vi "GettingStarted.vi"() -> ()   [LabVIEW 2014, in "Sixpack - Driver.lvlib"]
uses:
  Sixpack - Driver.lvlib
  Activity.ctl
  MotorParameter_P5.ctl
  MotorParameter_P6.ctl
  Current.ctl
panel:
  out "polling chart":u32(graph)
  out "error chart":i8(graph)
  in  "UnitAddress":u16=1
  out "error out":errorcluster
  out "StopFlag":bool
  out "CurrentActivity":T1
  out "CurrentPosition":i32 caption="Steps"
  out "Polling Time":u32 caption="msec"
  in  "Stop":bool
  in  "Tab Control":T2(tab)=enum."Interface"
  in  "Stop Motors":bool
  in  "Motors":T3
  in  "SetActualPos":bool
  in  "ActualPosition":u8 caption="Steps"
  in  "TargetPosition":i32 caption="Steps"
  in  "Ramp":bool
  out "TtlIo1":u8
  out "RefInput":bool
  out "AnalogInput":dbl(graph)
  out "AllInputs":T4
  in  "AcceleratingCurrent(100%)":T5
  in  "RunningCurrent(75%)":T5=enum."75%"
  in  "StandingCurrent(50%)":T5=enum."50%"
  in  "PowerDownCurrent(0%)":T5=enum."0%"
  in  "MotNr (0+1)":enum8{"0+1", "2+3", "4+5"}(ring)
  in  "Imax (0-800mA)":dbl=400.0
  in  "PowerDownDelay(500)":u16=500
  in  "SetCurrent":bool
  out "FMin":dbl
  out "FStart":dbl
  out "Fmax":dbl
  in  "VMax(511)":u16=511
  in  "AMax(128)":u16=128
  in  "Div(2)":u8=2
  in  "VMin(4)":u16=4
  in  "VStart(5)":u16=5
  in  "ClockDivider (5)":u8=5
  in  "SetVelocity":bool
  in  "PosLimit(6400)":u32=6400
  in  "SetMotorParameter":bool
  in  "P6 Bits":T6={"MT_OPTIMIZEWAY"=FALSE, "MT_FASTREF"=TRUE, "MT_MECHREF"=FALSE, "MT_DELAYTESTNULL"=TRUE, "MT_STOPSOFT"=FALSE, "MT_STOPNOREF"=FALSE, "MT_NULLPOSITIVE"=FALSE, "MUT_STOPFULSTEPS"=FALSE}
  in  "P5 Bits":T7={"MT_PI"=FALSE, "MT_ROTARY"=FALSE, "MT_AUTONULLCMD"=FALSE, "MT_TESTNULL"=FALSE, "MT_NULLLEFT"=FALSE, "MT_NULLCENTRE"=TRUE, "MT_STOPNULL"=FALSE, "MT_FILTERSWITCH"=TRUE}
  in  "SetLimits":bool
  in  "MaxRight(1023)":u16=1023
  in  "MinLeft(0)":u16
  in  "StartRefSearch":bool
  in  "Set ReferenceSwitchConfig":bool
  in  "Margin(0)":u16
  in  "TestNullRange(240)":u16
  in  "NullOffset(0)":i32
  out "FRefMax":dbl
  in  "DebouncingTime (22ms)":u8 format="%x"
  in  "VRefMax(100)":u16=100
  in  "Set RefSearchParameters":bool
  in  "Reset":bool
  out "SerialNumber":u16
  out "Temperature":i16 caption="Celsius"
  out "ResetFlag":bool
  out "FirmwareRevision":u8
  in  "OpenPort":bool
  out "Handle":i32=-1
  in  "BaudRate (19200)":enum32{"9600", "19200", "38400", "57600"}(ring)=enum."57600"
  in  "COM Port (COM1)":T8(ring)=enum."COM2"
  in  "MotNr":u8=1
  in  "PdcInt":i32=100 caption="msec"
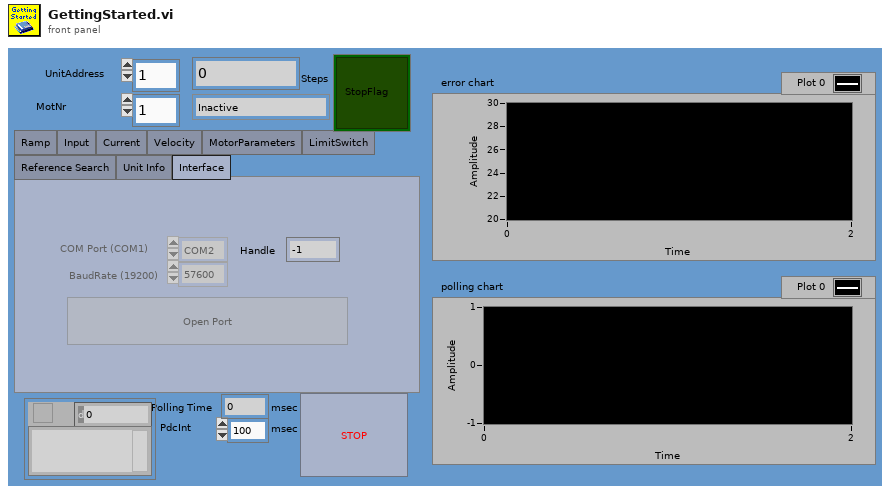
[diagram p1: front panel]
types:
  T1 = typedef "Sixpack - Driver.lvlib/Activity.ctl" = enum16{"Inactive", "Ramp", "PI-Controller", "Rotation", "ReferenceSearch", "Reference Search", "MechanicalReference"}
  T2 = enum32{"Ramp", "Input", "Current", "Velocity", "MotorParameters", "LimitSwitch", "Reference Search", "Unit Info", "Interface"}
  T3 = cluster{"Motor0":bool, "Motor1":bool, "Motor2":bool, "Motor3":bool, "Motor4":bool, "Motor5":bool}
  T4 = cluster{"Motor0":bool, "Motor1":bool, "Motor2":bool, "Motor3":bool, "Motor4":bool, "Motor5":bool, "Jumper1":bool, "Jumper2":bool}
  T5 = typedef "Sixpack - Driver.lvlib/Current.ctl" = enum8{"100%", "75%", "50%", "38%", "25%", "19%", "13%", "9%", "0%"}
  T6 = typedef "Sixpack - Driver.lvlib/MotorParameter_P6.ctl" = cluster{"MT_OPTIMIZEWAY":bool, "MT_FASTREF":bool, "MT_MECHREF":bool, "MT_DELAYTESTNULL":bool, "MT_STOPSOFT":bool, "MT_STOPNOREF":bool, "MT_NULLPOSITIVE":bool, "MUT_STOPFULSTEPS":bool}
  T7 = typedef "Sixpack - Driver.lvlib/MotorParameter_P5.ctl" = cluster{"MT_PI":bool, "MT_ROTARY":bool, "MT_AUTONULLCMD":bool, "MT_TESTNULL":bool, "MT_NULLLEFT":bool, "MT_NULLCENTRE":bool, "MT_STOPNULL":bool, "MT_FILTERSWITCH":bool}
  T8 = enum32{"COM1", "COM2", "COM3", "COM4", "COM5", "COM6", "COM7", "COM8", "COM9"}
  T9 = cluster{"MT_PI":bool, "MT_ROTARY":bool, "MT_AUTONULLCMD":bool, "MT_TESTNULL":bool, "MT_NULLLEFT":bool, "MT_NULLCENTRE":bool, "MT_STOPNULL":bool, "MT_FILTERSWITCH":bool}
  T10 = cluster{"MT_OPTIMIZEWAY":bool, "MT_FASTREF":bool, "MT_MECHREF":bool, "MT_DELAYTESTNULL":bool, "MT_STOPSOFT":bool, "MT_STOPNOREF":bool, "MT_NULLPOSITIVE":bool, "MUT_STOPFULSTEPS":bool}
  T11 = typedef "Sixpack.lvlib/Activity.ctl" = enum16{"Inactive", "Ramp", "PI-Controller", "Rotation", "ReferenceSearch", "Reference Search", "MechanicalReference"}
  T12 = typedef "Sixpack.lvlib/Current.ctl" = enum8{"100%", "75%", "50%", "38%", "25%", "19%", "13%", "9%", "0%"}
  T13 = typedef "Sixpack.lvlib/MotorParameter_P5.ctl" = cluster{"MT_PI":bool, "MT_ROTARY":bool, "MT_AUTONULLCMD":bool, "MT_TESTNULL":bool, "MT_NULLLEFT":bool, "MT_NULLCENTRE":bool, "MT_STOPNULL":bool, "MT_FILTERSWITCH":bool}
  T14 = typedef "Sixpack.lvlib/MotorParameter_P6.ctl" = cluster{"MT_OPTIMIZEWAY":bool, "MT_FASTREF":bool, "MT_MECHREF":bool, "MT_DELAYTESTNULL":bool, "MT_STOPSOFT":bool, "MT_STOPNOREF":bool, "MT_NULLPOSITIVE":bool, "MUT_STOPFULSTEPS":bool}
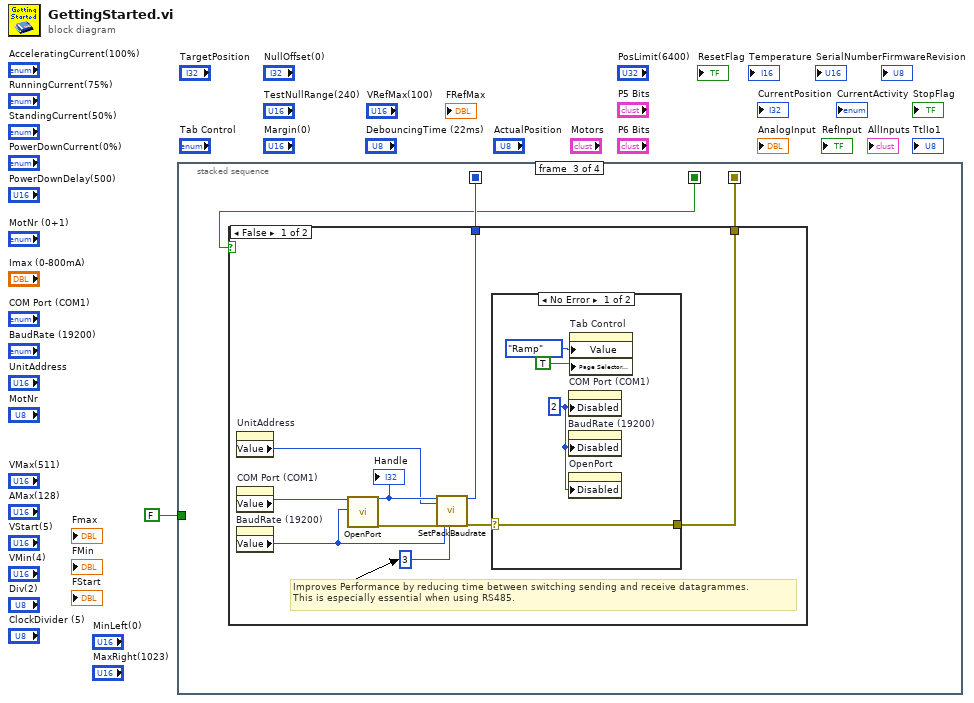
[diagram p0: block diagram]
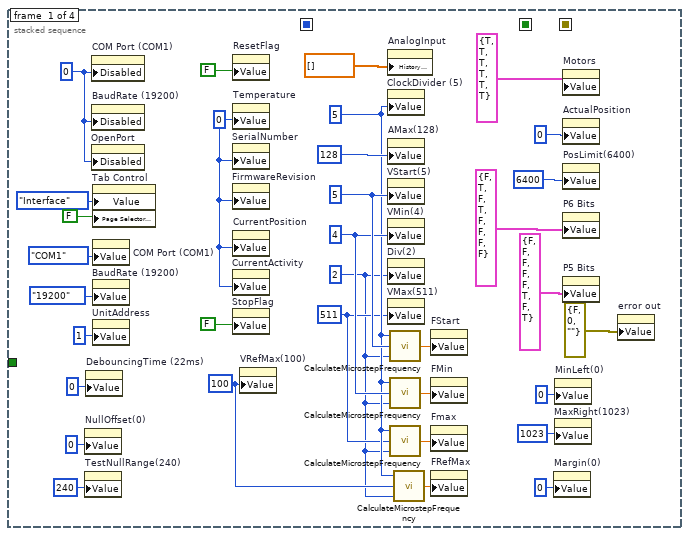
[diagram p2: hidden frame]
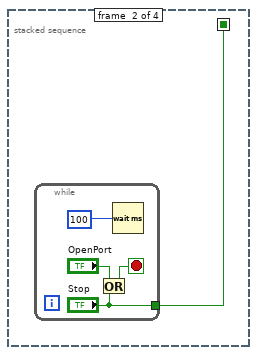
[diagram p3: hidden frame]
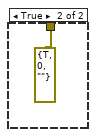
[diagram p5: hidden frame]
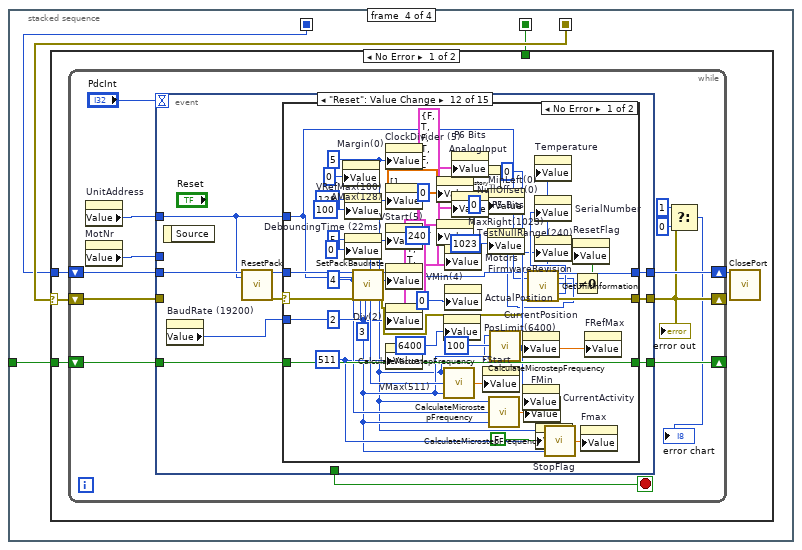
[diagram p6: hidden frame]
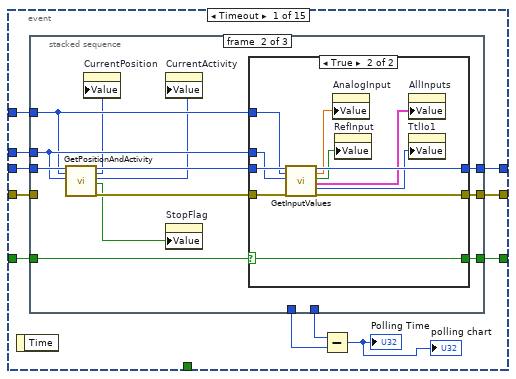
[diagram p7: hidden frame]
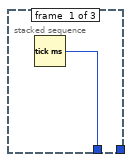
[diagram p8: hidden frame]
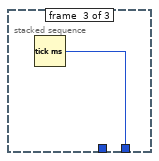
[diagram p10: hidden frame]
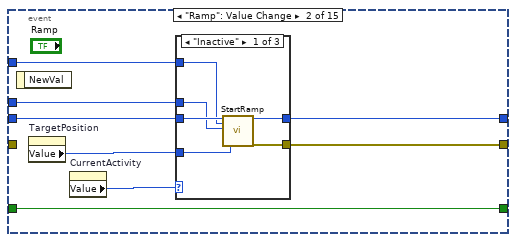
[diagram p11: hidden frame]
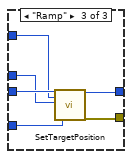
[diagram p13: hidden frame]
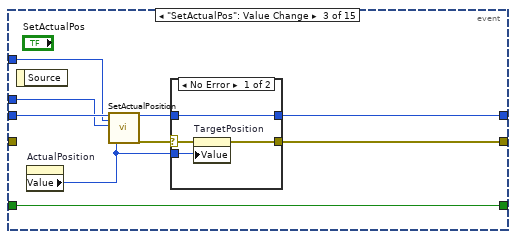
[diagram p14: hidden frame]
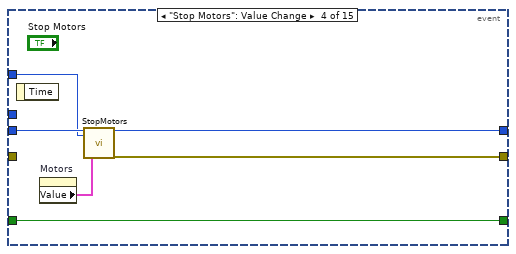
[diagram p16: hidden frame]
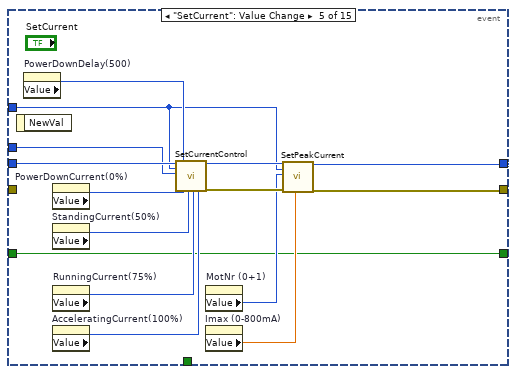
[diagram p17: hidden frame]
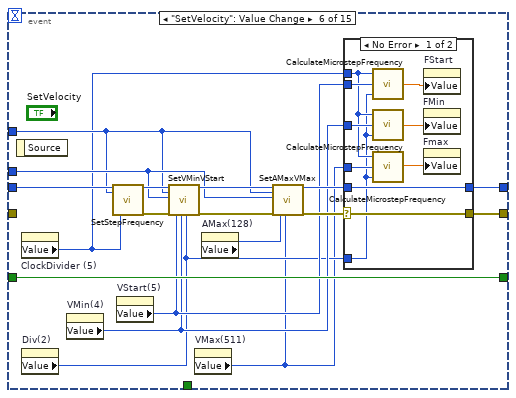
[diagram p18: hidden frame]
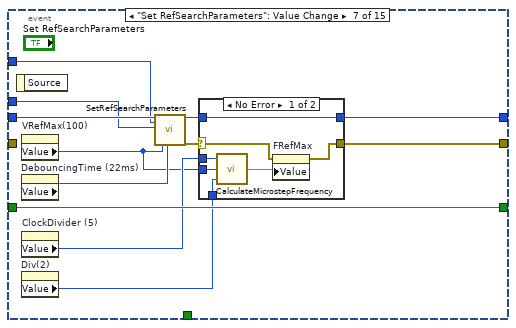
[diagram p20: hidden frame]
diagram:
  n1 = stacked-sequence {
    seq-local: [_ _ w42 _] -> [_ _ _ w60]
    seq-local: [_ _ w41 _] -> [_ _ _ w59]
    seq-local: [_ w35 _ _] -> [_ _ w40 w58]
    tunnel: FALSE ("ReadInput") -> [_ _ _ w61]
    frame #0 {
      w12 = u16 100 ("VRefMax(100)")
      w10 = u16 511 ("VMax(511)")
      w2 = u8 2 ("Div(2)")
      w20 = u16 4 ("VMin(4)")
      w21 = u16 5 ("VStart(5)")
      w11 = u8 5 ("ClockDivider (5)")
      w23 = i16 0 ("Temperature")
      w33 = u8 0 ("Disabled")
      n2 = property on="NullOffset(0)" class="DigNum (strict)"("Value"=0 ("NullOffset(0)")) -> ()  [unwired: 2 in, 2 out]
      n3 = property on="TestNullRange(240)" class="DigNum (strict)"("Value"=u16 240 ("TestNullRange(240)")) -> ()  [unwired: 2 in, 2 out]
      n4 = property on="DebouncingTime (22ms)" class="DigNum (strict)"("Value"=u16 0 ("DebouncingTime (22ms)")) -> ()  [unwired: 2 in, 2 out]
      n5 = property on="COM Port (COM1)" class="Enum (strict)"("Disabled"=w33) -> ()  [unwired: 2 in, 2 out]
      n6 = property on="BaudRate (19200)" class="Enum (strict)"("Disabled"=w33) -> ()  [unwired: 2 in, 2 out]
      n7 = property on="OpenPort" class="Bool"("Disabled"=w33) -> ()  [unwired: 2 in, 2 out]
      n8 = property on="Tab Control" class="TabCtl (strict)"("Value"=T2."Interface" ("Tab Control"), "Page Selector Visible"=FALSE) -> ()  [unwired: 2 in, 2 out]
      n9 = property on="COM Port (COM1)" class="Enum (strict)"("Value"=T8."COM1" ("COM Port (COM1)")) -> ()  [unwired: 2 in, 2 out]
      n10 = property on="BaudRate (19200)" class="Enum (strict)"("Value"=enum32{"9600", "19200", "38400", "57600"}."19200" ("BaudRate (19200)")) -> ()  [unwired: 2 in, 2 out]
      n11 = property on="UnitAddress" class="DigNum (strict)"("Value"=u16 1 ("UnitAddress")) -> ()  [unwired: 2 in, 2 out]
      n12 = property on="ResetFlag" class="Bool (strict)"("Value"=FALSE ("ResetFlag")) -> ()  [unwired: 2 in, 2 out]
      n13 = property on="Temperature" class="DigNum (strict)"("Value"=w23) -> ()  [unwired: 2 in, 2 out]
      n14 = property on="SerialNumber" class="DigNum (strict)"("Value"=w23) -> ()  [unwired: 2 in, 2 out]
      n15 = property on="FirmwareRevision" class="DigNum (strict)"("Value"=w23) -> ()  [unwired: 2 in, 2 out]
      n16 = property on="CurrentPosition" class="DigNum (strict)"("Value"=w23) -> ()  [unwired: 2 in, 2 out]
      n17 = property on="CurrentActivity" class="Enum (strict)"("Value"=w23) -> ()  [unwired: 2 in, 2 out]
      n18 = property on="StopFlag" class="Bool (strict)"("Value"=FALSE ("StopFlag")) -> ()  [unwired: 2 in, 2 out]
      n19 = property on="VRefMax(100)" class="DigNum (strict)"("Value"=w12) -> ()  [unwired: 2 in, 2 out]
      n20 = property on="AnalogInput" class="WFChart (strict)"("History Data"=dbl[] []) -> ()  [unwired: 2 in, 2 out]
      n21 = property on="ClockDivider (5)" class="DigNum (strict)"("Value"=w11) -> ()  [unwired: 2 in, 2 out]
      n22 = property on="AMax(128)" class="DigNum (strict)"("Value"=u16 128 ("AMax(128)")) -> ()  [unwired: 2 in, 2 out]
      n23 = property on="VStart(5)" class="DigNum (strict)"("Value"=w21) -> ()  [unwired: 2 in, 2 out]
      n24 = property on="VMin(4)" class="DigNum (strict)"("Value"=w20) -> ()  [unwired: 2 in, 2 out]
      n25 = property on="Div(2)" class="DigNum (strict)"("Value"=w2) -> ()  [unwired: 2 in, 2 out]
      n26 = property on="VMax(511)" class="DigNum (strict)"("Value"=w10) -> ()  [unwired: 2 in, 2 out]
      n27 = call "CalculateMicrostepFrequency.vi"("div_i"=w2, "velocity"=w21, "clkdiv"=w11) -> ("f_microstep"=w27:dbl)
      n28 = call "CalculateMicrostepFrequency.vi"("div_i"=w2, "velocity"=w20, "clkdiv"=w11) -> ("f_microstep"=w26:dbl)
      n29 = call "CalculateMicrostepFrequency.vi"("div_i"=w2, "velocity"=w10, "clkdiv"=w11) -> ("f_microstep"=w25:dbl)
      n30 = call "CalculateMicrostepFrequency.vi"("div_i"=w2, "velocity"=w12, "clkdiv"=w11) -> ("f_microstep"=w13:dbl)
      n31 = property on="FStart" class="DigNum (strict)"("Value"=w27) -> ()  [unwired: 2 in, 2 out]
      n32 = property on="FMin" class="DigNum (strict)"("Value"=w26) -> ()  [unwired: 2 in, 2 out]
      n33 = property on="Fmax" class="DigNum (strict)"("Value"=w25) -> ()  [unwired: 2 in, 2 out]
      n34 = property on="FRefMax" class="DigNum (strict)"("Value"=w13) -> ()  [unwired: 2 in, 2 out]
      n35 = property on="Margin(0)" class="DigNum (strict)"("Value"=u16 0 ("Margin(0)")) -> ()  [unwired: 2 in, 2 out]
      n36 = property on="MinLeft(0)" class="DigNum (strict)"("Value"=u16 0 ("MinLeft(0)")) -> ()  [unwired: 2 in, 2 out]
      n37 = property on="MaxRight(1023)" class="DigNum (strict)"("Value"=u16 1023 ("MaxRight(1023)")) -> ()  [unwired: 2 in, 2 out]
      n38 = property on="Motors" class="Clust (strict)"("Value"=T3 {"Motor0"=TRUE, "Motor1"=TRUE, "Motor2"=TRUE, "Motor3"=TRUE, "Motor4"=TRUE, "Motor5"=TRUE} ("Motors")) -> ()  [unwired: 2 in, 2 out]
      n39 = property on="ActualPosition" class="DigNum (strict)"("Value"=u8 0 ("ActualPosition")) -> ()  [unwired: 2 in, 2 out]
      n40 = property on="PosLimit(6400)" class="DigNum (strict)"("Value"=u32 6400 ("PosLimit(6400)")) -> ()  [unwired: 2 in, 2 out]
      n41 = property on="P6 Bits" class="Clust (strict)"("Value"=T10 {"MT_OPTIMIZEWAY"=FALSE, "MT_FASTREF"=TRUE, "MT_MECHREF"=FALSE, "MT_DELAYTESTNULL"=TRUE, "MT_STOPSOFT"=FALSE, "MT_STOPNOREF"=FALSE, "MT_NULLPOSITIVE"=FALSE, "MUT_STOPFULSTEPS"=FALSE}) -> ()  [unwired: 2 in, 2 out]
      n42 = property on="P5 Bits" class="Clust (strict)"("Value"=T9 {"MT_PI"=FALSE, "MT_ROTARY"=FALSE, "MT_AUTONULLCMD"=FALSE, "MT_TESTNULL"=FALSE, "MT_NULLLEFT"=FALSE, "MT_NULLCENTRE"=TRUE, "MT_STOPNULL"=FALSE, "MT_FILTERSWITCH"=TRUE}) -> ()  [unwired: 2 in, 2 out]
      n43 = property on="error out" class="Clust (strict)"("Value"=errorcluster {"status"=FALSE, "code"=0, "source"=""} ("error out")) -> ()  [unwired: 2 in, 2 out]
    }
    frame #1 {
      n44 = while {
        tunnel: ["Stop"] -> w35
        stop <- w38 stop-if-true
        n45 = Or(x="OpenPort", y="Stop") -> (x .or. y?=w38:bool)
        n46 = Wait (ms)(milliseconds to wait=100) -> ()  [unwired: 1 out]
      }
    }
    frame #2 {
      n47 = case shown="False" w40 {
        tunnel: [w47 errorcluster {"status"=TRUE, "code"=0, "source"=""} ("error IO")] -> w42
        tunnel: [w46 _] -> w41
        frame False {
          # "Improves Performance by reducing time between switching sending and receive datagrammes.\nThis is especially essential when using RS485."
          n48 = property on="UnitAddress" class="DigNum (strict)"() -> ("Value"=w43:u16)  [unwired: 2 in, 2 out]
          n49 = property on="COM Port (COM1)" class="Enum (strict)"() -> ("Value"=w45:T8)  [unwired: 2 in, 2 out]
          n50 = property on="BaudRate (19200)" class="Enum (strict)"() -> ("Value"=w44:enum32{"9600", "19200", "38400", "57600"})  [unwired: 2 in, 2 out]
          n51 = call "OpenPort.vi"("COM Port (COM1)"=w45, "BaudRate (19200)"=w44) -> ("handle"=w50:i32, "error out"=w49:errorcluster)  [unwired: 16 in]
          "Handle" <- w50
          n52 = call "SetPackBaudrate.vi"("handle in"=w50, "UnitAddress(0)"=w43, "error in"=w49, "BaudRate (19200)"=w44, "Delay(6)"=u16 3 ("Delay")) -> ("handle out"=w46:i32, "error out"=w48:errorcluster)  [unwired: 13 in]
          n53 = case shown="No Error" w48 {
            selector: w48 -> [w55 w56]
            tunnel: [w55 w56] -> w47
            frame No Error {
              w53 = u8 2 ("Disabled")
              n54 = property on="COM Port (COM1)" class="Enum (strict)"("Disabled"=w53) -> ()  [unwired: 2 in, 2 out]
              n55 = property on="BaudRate (19200)" class="Enum (strict)"("Disabled"=w53) -> ()  [unwired: 2 in, 2 out]
              n56 = property on="OpenPort" class="Bool"("Disabled"=w53) -> ()  [unwired: 2 in, 2 out]
              n57 = property on="Tab Control" class="TabCtl (strict)"("Value"=T2."Ramp" ("Tab Control"), "Page Selector Visible"=TRUE) -> ()  [unwired: 2 in, 2 out]
            }
            frame Error {
            }
          }
        }
        frame True {
        }
      }
    }
    frame #3 {
      n58 = case shown="No Error" w60 {
        selector: w60 -> [w63 w336]
        tunnel: w61 -> [w65 _]
        tunnel: w59 -> [w62 _]
        tunnel: w58 -> [_ w335]
        frame No Error {
          n59 = while {
            shift-right: [w70] -> w64
            shift-left: w62 -> [w78]
            shift-right: [w74] -> _
            shift-left: w65 -> [w75]
            shift-right: [w69] -> _
            shift-left: w63 -> [w73]
            stop <- w77 stop-if-true
            n60 = property on="UnitAddress" class="DigNum (strict)"() -> ("Value"=w71:u16)  [unwired: 2 in, 2 out]
            n61 = property on="MotNr" class="DigNum (strict)"() -> ("Value"=w72:u8)  [unwired: 2 in, 2 out]
            n62 = event shown="[11] \"Reset\": Value Change" {
              selector: _ -> [_ _ _ _ _ _ _ _ _ _ _ _ _ _ _]
              dyn-events: _ -> [_ _ _ _ _ _ _ _ _ _ _ _ _ _ _]
              timeout: "PdcInt" -> [_ _ _ _ _ _ _ _ _ _ _ _ _ _ _]
              tunnel: w78 -> [w89 w125 w147 w159 w174 w192 w213 w234 w244 w252 w258 w267 w316 w329 w333]
              tunnel: [w88 w124 w144 w158 w172 w184 w205 w226 w242 w247 w257 w265 w316 w329 w333] -> w70
              tunnel: [_ _ _ _ _ _ _ _ _ _ _ _ _ _ w334] -> w77
              tunnel: [w85 w123 w143 w157 w168 w183 w206 w230 w243 w248 w256 w263 w318 w327 w331] -> w69
              tunnel: w75 -> [w84 w120 w146 w156 w162 w187 w216 _ w241 _ w255 w259 _ w328 w332]
              tunnel: [w83 w120 w146 w156 w162 w187 w216 _ w241 _ w255 w260 w317 w328 w332] -> w74
              tunnel: w73 -> [w82 _ _ _ _ _ _ _ _ w251 _ _ _ w327 w331]
              tunnel: w72 -> [w81 w118 w139 _ w160 w182 w207 w233 w239 w249 w253 _ w314 _ _]
              tunnel: w71 -> [w80 w119 w140 w155 w161 w181 w208 w232 w240 w250 w254 w261 w315 _ _]
              event Timeout {
                n63 = event-data() -> ()  [unwired: 1 in, 1 out]
                n64 = stacked-sequence {
                  tunnel: w89 -> [_ w101 _]
                  tunnel: [w90 _ _] -> w86
                  tunnel: [_ _ w117] -> w87
                  tunnel: [_ w102 _] -> w88
                  tunnel: [_ w97 _] -> w85
                  tunnel: w84 -> [_ w96 _]
                  tunnel: [_ w95 _] -> w83
                  tunnel: w82 -> [_ _ _]
                  tunnel: w81 -> [_ w94 _]
                  tunnel: w80 -> [_ w93 _]
                  frame #0 {
                    n65 = Tick Count (ms)() -> (millisecond timer value=w90:u32)
                  }
                  frame #1 {
                    n66 = call "GetPositionAndActivity.vi"("handle in"=w101, "UnitAddress(0)"=w93, "MotNr(0)"=w94) -> ("handle out"=w100:i32, "CurrentPosition"=w91:i32, "CurrentActivity"=w92:T1, "StopFlag"=w98:bool, "error out"=w99:errorcluster)  [unwired: 12 in]
                    n67 = property on="CurrentPosition" class="DigNum (strict)"("Value"=w91) -> ()  [unwired: 2 in, 2 out]
                    n68 = property on="CurrentActivity" class="Enum (strict)"("Value"=w92) -> ()  [unwired: 2 in, 2 out]
                    n69 = property on="StopFlag" class="Bool (strict)"("Value"=w98) -> ()  [unwired: 2 in, 2 out]
                    n70 = case shown="True" w96 {
                      selector: w96 -> [w103 w112]
                      tunnel: w100 -> [w105 w116]
                      tunnel: [w105 w115] -> w102
                      tunnel: w99 -> [w104 w114]
                      tunnel: [w104 w113] -> w97
                      tunnel: [w103 w112] -> w95
                      tunnel: w93 -> [_ w107]
                      tunnel: w94 -> [_ w106]
                      frame False {
                      }
                      frame True {
                        n71 = call "GetInputValues.vi"("handle in"=w116, "UnitAddress(0)"=w107, "Channel(0)"=w106, "error in"=w114) -> ("handle out"=w115:i32, "AnalogueValue (V)"=w111:dbl, "RefInput"=w110:bool, "AllInputs"=w108:T4, "TtlIo1"=w109:u8, "error out"=w113:errorcluster)  [unwired: 10 in]
                        n72 = property on="AnalogInput" class="WFChart (strict)"("Value"=w111) -> ()  [unwired: 2 in, 2 out]
                        n73 = property on="RefInput" class="Bool (strict)"("Value"=w110) -> ()  [unwired: 2 in, 2 out]
                        n74 = property on="AllInputs" class="Clust (strict)"("Value"=w108) -> ()  [unwired: 2 in, 2 out]
                        n75 = property on="TtlIo1" class="DigNum (strict)"("Value"=w109) -> ()  [unwired: 2 in, 2 out]
                      }
                    }
                  }
                  frame #2 {
                    n76 = Tick Count (ms)() -> (millisecond timer value=w117:u32)
                  }
                }
                n77 = Subtract(x=w87, y=w86) -> (x-y=→"Polling Time" →"polling chart":u32)
              }
              event "Ramp": Value Change {
                n78 = event-data() -> ()  [unwired: 1 in, 1 out]
                n79 = property on="TargetPosition" class="DigNum (strict)"() -> ("Value"=w121:i32)  [unwired: 2 in, 2 out]
                n80 = property on="CurrentActivity" class="Enum (strict)"() -> ("Value"=w122:T11)  [unwired: 2 in, 2 out]
                n81 = case shown="\"Inactive\"" w122 {
                  tunnel: w125 -> [w131 w132 w138]
                  tunnel: [w130 w132 w137] -> w124
                  tunnel: w121 -> [w128 _ w135]
                  tunnel: [w129 _ w136] -> w123
                  tunnel: w119 -> [w127 _ w134]
                  tunnel: w118 -> [w126 _ w133]
                  frame "Inactive" {
                    n82 = call "StartRamp.vi"("handle in"=w131, "UnitAddress(0)"=w127, "MotNr(0)"=w126, "TargetPosition(0)"=w128) -> ("handle out"=w130:i32, "error out"=w129:errorcluster)  [unwired: 14 in]
                  }
                  frame Default {
                  }
                  frame "Ramp" {
                    n83 = call "SetTargetPosition.vi"("handle in"=w138, "UnitAddress(0)"=w134, "MotNr(0)"=w133, "TargetPosition(0)"=w135) -> ("handle out"=w137:i32, "error out"=w136:errorcluster)  [unwired: 14 in]
                  }
                }
              }
              event "SetActualPos": Value Change {
                n84 = event-data() -> ()  [unwired: 1 in, 1 out]
                n85 = property on="ActualPosition" class="DigNum (strict)"() -> ("Value"=w141:u8)  [unwired: 2 in, 2 out]
                n86 = call "SetActualPosition.vi"("handle in"=w147, "UnitAddress(0)"=w140, "MotNr(0)"=w139, "ActualPosition(0)"=w141) -> ("handle out"=w145:i32, "error out"=w142:errorcluster)  [unwired: 14 in]
                n87 = case shown="No Error" w142 {
                  selector: w142 -> [w151 w152]
                  tunnel: w145 -> [w148 w153]
                  tunnel: [w148 w153] -> w144
                  tunnel: [w150 w152] -> w143
                  tunnel: w141 -> [w149 _]
                  frame No Error {
                    n88 = property on="TargetPosition" class="DigNum (strict)"(error in=w151, "Value"=w149) -> (error out=w150:errorcluster)  [unwired: 1 in, 1 out]
                  }
                  frame Error {
                  }
                }
              }
              event "Stop Motors": Value Change {
                n89 = event-data() -> ()  [unwired: 1 in, 1 out]
                n90 = property on="Motors" class="Clust (strict)"() -> ("Value"=w154:T3)  [unwired: 2 in, 2 out]
                n91 = call "StopMotors.vi"("handle in"=w159, "UnitAddress(0)"=w155, "Motors"=w154) -> ("handle out"=w158:i32, "error out"=w157:errorcluster)  [unwired: 15 in]
              }
              event "SetCurrent": Value Change {
                n92 = event-data() -> ()  [unwired: 1 in, 1 out]
                n93 = property on="PowerDownDelay(500)" class="DigNum (strict)"() -> ("Value"=w165:u16)  [unwired: 2 in, 2 out]
                n94 = property on="PowerDownCurrent(0%)" class="Enum (strict)"() -> ("Value"=w171:T12)  [unwired: 2 in, 2 out]
                n95 = property on="StandingCurrent(50%)" class="Enum (strict)"() -> ("Value"=w170:T12)  [unwired: 2 in, 2 out]
                n96 = property on="RunningCurrent(75%)" class="Enum (strict)"() -> ("Value"=w167:T12)  [unwired: 2 in, 2 out]
                n97 = property on="AcceleratingCurrent(100%)" class="Enum (strict)"() -> ("Value"=w166:T12)  [unwired: 2 in, 2 out]
                n98 = call "SetCurrentControl.vi"("handle in"=w174, "UnitAddress(0)"=w161, "MotNr(0)"=w160, 6:w165, "I Control"=w171, 9:w170, 11:w167, 13:w166) -> ("handle out"=w173:i32, "error out"=w169:errorcluster)  [unwired: 10 in]
                n99 = property on="MotNr (0+1)" class="Enum (strict)"() -> ("Value"=w163:enum8{"0+1", "2+3", "4+5"})  [unwired: 2 in, 2 out]
                n100 = property on="Imax (0-800mA)" class="DigNum (strict)"() -> ("Value"=w164:dbl)  [unwired: 2 in, 2 out]
                n101 = call "SetPeakCurrent.vi"("handle in"=w173, "UnitAddress (0)"=w161, "MotNr (0+1)"=w163, "error in(no error)"=w169, "Imax (50%)"=w164) -> ("handle out"=w172:i32, "error out"=w168:errorcluster)  [unwired: 13 in]
              }
              event "SetVelocity": Value Change {
                n102 = event-data() -> ()  [unwired: 1 in, 1 out]
                n103 = property on="ClockDivider (5)" class="DigNum (strict)"() -> ("Value"=w179:u8)  [unwired: 2 in, 2 out]
                n104 = property on="Div(2)" class="DigNum (strict)"() -> ("Value"=w177:u8)  [unwired: 2 in, 2 out]
                n105 = property on="VMin(4)" class="DigNum (strict)"() -> ("Value"=w178:u16)  [unwired: 2 in, 2 out]
                n106 = call "SetStepFrequency.vi"("handle in"=w192, "UnitAddress(0)"=w181, "ClockDivider (5)"=w179) -> ("handle out"=w191:i32, "error out"=w189:errorcluster)  [unwired: 15 in]
                n107 = property on="VStart(5)" class="DigNum (strict)"() -> ("Value"=w180:u16)  [unwired: 2 in, 2 out]
                n108 = call "SetVMinVStart.vi"("handle in"=w191, "UnitAddress(0)"=w181, "MotNr(0)"=w182, "error in"=w189, "VminVStart"=w180, 9:w178, 11:w177) -> ("handle out"=w190:i32, "error out"=w188:errorcluster)  [unwired: 11 in]
                n109 = property on="VMax(511)" class="DigNum (strict)"() -> ("Value"=w176:u16)  [unwired: 2 in, 2 out]
                n110 = property on="AMax(128)" class="DigNum (strict)"() -> ("Value"=w175:u16)  [unwired: 2 in, 2 out]
                n111 = call "SetAMaxVMax.vi"("handle in"=w190, "UnitAddress(0)"=w181, "MotNr(0)"=w182, "error in"=w188, "VMaxAMax"=w175, 9:w176) -> ("handle out"=w185:i32, "error out"=w186:errorcluster)  [unwired: 12 in]
                n112 = case shown="No Error" w186 {
                  selector: w186 -> [w201 w203]
                  tunnel: w185 -> [w202 w204]
                  tunnel: [w202 w204] -> w184
                  tunnel: w179 -> [w198 _]
                  tunnel: [w201 w203] -> w183
                  tunnel: w180 -> [w200 _]
                  tunnel: w178 -> [w199 _]
                  tunnel: w176 -> [w197 _]
                  tunnel: w177 -> [w196 _]
                  frame No Error {
                    n113 = call "CalculateMicrostepFrequency.vi"("div_i"=w196, "velocity"=w200, "clkdiv"=w198) -> ("f_microstep"=w195:dbl)
                    n114 = call "CalculateMicrostepFrequency.vi"("div_i"=w196, "velocity"=w199, "clkdiv"=w198) -> ("f_microstep"=w194:dbl)
                    n115 = call "CalculateMicrostepFrequency.vi"("div_i"=w196, "velocity"=w197, "clkdiv"=w198) -> ("f_microstep"=w193:dbl)
                    n116 = property on="FStart" class="DigNum (strict)"("Value"=w195) -> ()  [unwired: 2 in, 2 out]
                    n117 = property on="FMin" class="DigNum (strict)"("Value"=w194) -> ()  [unwired: 2 in, 2 out]
                    n118 = property on="Fmax" class="DigNum (strict)"("Value"=w193) -> ()  [unwired: 2 in, 2 out]
                  }
                  frame Error {
                  }
                }
              }
              event "Set RefSearchParameters": Value Change {
                n119 = event-data() -> ()  [unwired: 1 in, 1 out]
                n120 = property on="VRefMax(100)" class="DigNum (strict)"() -> ("Value"=w209:u16)  [unwired: 2 in, 2 out]
                n121 = property on="DebouncingTime (22ms)" class="DigNum (strict)"() -> ("Value"=w210:u8)  [unwired: 2 in, 2 out]
                n122 = property on="ClockDivider (5)" class="DigNum (strict)"() -> ("Value"=w215:u8)  [unwired: 2 in, 2 out]
                n123 = property on="Div(2)" class="DigNum (strict)"() -> ("Value"=w214:u8)  [unwired: 2 in, 2 out]
                n124 = call "SetRefSearchParameters.vi"("handle in"=w213, "UnitAddress(0)"=w208, "MotNr(0)"=w207, "Ref Search Parameter"=w209, 9:w210) -> ("handle out"=w212:i32, "error out"=w211:errorcluster)  [unwired: 13 in]
                n125 = case shown="No Error" w211 {
                  selector: w211 -> [w218 w225]
                  tunnel: [w217 w225] -> w206
                  tunnel: [w223 w224] -> w205
                  tunnel: w212 -> [w223 w224]
                  tunnel: w215 -> [w222 _]
                  tunnel: w209 -> [w221 _]
                  tunnel: w214 -> [w220 _]
                  frame No Error {
                    n126 = call "CalculateMicrostepFrequency.vi"("div_i"=w220, "velocity"=w221, "clkdiv"=w222) -> ("f_microstep"=w219:dbl)
                    n127 = property on="FRefMax" class="DigNum (strict)"(error in=w218, "Value"=w219) -> (error out=w217:errorcluster)  [unwired: 1 in, 1 out]
                  }
                  frame Error {
                  }
                }
              }
              event "Set ReferenceSwitchConfig": Value Change {
                n128 = event-data() -> ()  [unwired: 1 in, 1 out]
                n129 = property on="NullOffset(0)" class="DigNum (strict)"() -> ("Value"=w229:i32)  [unwired: 2 in, 2 out]
                n130 = property on="TestNullRange(240)" class="DigNum (strict)"() -> ("Value"=w228:u16)  [unwired: 2 in, 2 out]
                n131 = property on="Margin(0)" class="DigNum (strict)"() -> ("Value"=w227:u16)  [unwired: 2 in, 2 out]
                n132 = call "SetNullPointOffset.vi"("handle in"=w234, "UnitAddress(0)"=w232, "MotNr(0)"=w233, "NullOffset(0)"=w229, "TestNullRange(240)"=w228) -> ("handle out"=w235:i32, "error out"=w231:errorcluster)  [unwired: 13 in]
                n133 = call "SetMargin.vi"("handle in"=w235, "UnitAddress(0)"=w232, "MotNr(0..5)"=w233, "error in"=w231, "Margin(0)"=w227) -> ("handle out"=w226:i32, "error out"=w230:errorcluster)  [unwired: 13 in]
              }
              event "SetMotorParameter": Value Change {
                n134 = event-data() -> ()  [unwired: 1 in, 1 out]
                n135 = property on="PosLimit(6400)" class="DigNum (strict)"() -> ("Value"=w238:u32)  [unwired: 2 in, 2 out]
                n136 = property on="P5 Bits" class="Clust (strict)"() -> ("Value"=w237:T13)  [unwired: 2 in, 2 out]
                n137 = property on="P6 Bits" class="Clust (strict)"() -> ("Value"=w236:T14)  [unwired: 2 in, 2 out]
                n138 = call "SetMotorParameters.vi"("handle in"=w244, "UnitAddress(0)"=w240, "MotNr(0)"=w239, "Motor Parameter"=w238, 9:w237, 11:w236) -> ("handle out"=w242:i32, "error out"=w243:errorcluster)  [unwired: 12 in]
              }
              event "SetLimits": Value Change {
                n139 = event-data() -> ()  [unwired: 1 in, 1 out]
                n140 = property on="MinLeft(0)" class="DigNum (strict)"() -> ("Value"=w246:u16)  [unwired: 2 in, 2 out]
                n141 = property on="MaxRight(1023)" class="DigNum (strict)"() -> ("Value"=w245:u16)  [unwired: 2 in, 2 out]
                n142 = call "SetStopSwitchLimits.vi"("handle in"=w252, "UnitAddress(0)"=w250, "Channel(0)"=w249, "error in"=w251, "Stopswitch Limits"=w246, 9:w245) -> ("handle out"=w247:i32, "error out"=w248:errorcluster)  [unwired: 12 in]
              }
              event "StartRefSearch": Value Change {
                n143 = event-data() -> ()  [unwired: 1 in, 1 out]
                n144 = call "ReferenceSearch.vi"("handle in"=w258, "UnitAddress(0)"=w254, "MotNr(0)"=w253) -> ("handle out"=w257:i32, "error out"=w256:errorcluster)  [unwired: 15 in]
              }
              event "Reset": Value Change {
                n145 = event-data() -> ()  [unwired: 1 in, 1 out]
                n146 = property on="BaudRate (19200)" class="Enum (strict)"() -> ("Value"=w262:enum32{"9600", "19200", "38400", "57600"})  [unwired: 2 in, 2 out]
                n147 = call "ResetPack.vi"("handle in"=w267, "UnitAddress(0)"=w261) -> ("handle out"=w264:i32, "error out"=w266:errorcluster)  [unwired: 16 in]
                n148 = case shown="No Error" w266 {
                  selector: w266 -> [w268 w310]
                  tunnel: [w287 w311] -> w265
                  tunnel: w264 -> [w306 w311]
                  tunnel: [w286 w310] -> w263
                  tunnel: w262 -> [w307 _]
                  tunnel: w261 -> [w285 _]
                  tunnel: [w305 w309] -> w260
                  tunnel: w259 -> [w305 w309]
                  frame No Error {
                    w288 = u16 511 ("VMax(511)")
                    w276 = u8 2 ("Div(2)")
                    w289 = u16 4 ("VMin(4)")
                    w290 = u16 5 ("VStart(5)")
                    w269 = u8 5 ("ClockDivider (5)")
                    w301 = i16 0 ("Temperature")
                    n149 = property on="Margin(0)" class="DigNum (strict)"("Value"=u16 0 ("Margin(0)")) -> ()  [unwired: 2 in, 2 out]
                    n150 = property on="VRefMax(100)" class="DigNum (strict)"("Value"=u16 100 ("VRefMax(100)")) -> ()  [unwired: 2 in, 2 out]
                    n151 = property on="DebouncingTime (22ms)" class="DigNum (strict)"("Value"=u16 0 ("DebouncingTime (22ms)")) -> ()  [unwired: 2 in, 2 out]
                    n152 = call "SetPackBaudrate.vi"("handle in"=w306, "UnitAddress(0)"=w285, "error in"=w268, "BaudRate (19200)"=w307, "Delay(6)"=u16 3 ("Delay")) -> ("handle out"=w284:i32, "error out"=w283:errorcluster)  [unwired: 13 in]
                    n153 = property on="ClockDivider (5)" class="DigNum (strict)"("Value"=w269) -> ()  [unwired: 2 in, 2 out]
                    n154 = property on="AMax(128)" class="DigNum (strict)"("Value"=u16 128 ("AMax(128)")) -> ()  [unwired: 2 in, 2 out]
                    n155 = property on="VStart(5)" class="DigNum (strict)"("Value"=w290) -> ()  [unwired: 2 in, 2 out]
                    n156 = property on="VMin(4)" class="DigNum (strict)"("Value"=w289) -> ()  [unwired: 2 in, 2 out]
                    n157 = property on="Div(2)" class="DigNum (strict)"("Value"=w276) -> ()  [unwired: 2 in, 2 out]
                    n158 = property on="VMax(511)" class="DigNum (strict)"("Value"=w288) -> ()  [unwired: 2 in, 2 out]
                    n159 = property on="NullOffset(0)" class="DigNum (strict)"("Value"=0 ("NullOffset(0)")) -> ()  [unwired: 2 in, 2 out]
                    n160 = property on="TestNullRange(240)" class="DigNum (strict)"("Value"=u16 240 ("TestNullRange(240)")) -> ()  [unwired: 2 in, 2 out]
                    n161 = property on="PosLimit(6400)" class="DigNum (strict)"("Value"=u32 6400 ("PosLimit(6400)")) -> ()  [unwired: 2 in, 2 out]
                    n162 = call "CalculateMicrostepFrequency.vi"("div_i"=w276, "velocity"=w290, "clkdiv"=w269) -> ("f_microstep"=w294:dbl)
                    n163 = property on="Motors" class="Clust (strict)"("Value"=T3 {"Motor0"=TRUE, "Motor1"=TRUE, "Motor2"=TRUE, "Motor3"=TRUE, "Motor4"=TRUE, "Motor5"=TRUE} ("Motors")) -> ()  [unwired: 2 in, 2 out]
                    n164 = property on="ActualPosition" class="DigNum (strict)"("Value"=u8 0 ("ActualPosition")) -> ()  [unwired: 2 in, 2 out]
                    n165 = property on="P6 Bits" class="Clust (strict)"("Value"=T10 {"MT_OPTIMIZEWAY"=FALSE, "MT_FASTREF"=TRUE, "MT_MECHREF"=FALSE, "MT_DELAYTESTNULL"=TRUE, "MT_STOPSOFT"=FALSE, "MT_STOPNOREF"=FALSE, "MT_NULLPOSITIVE"=FALSE, "MUT_STOPFULSTEPS"=FALSE}) -> ()  [unwired: 2 in, 2 out]
                    n166 = property on="P5 Bits" class="Clust (strict)"("Value"=T9 {"MT_PI"=FALSE, "MT_ROTARY"=FALSE, "MT_AUTONULLCMD"=FALSE, "MT_TESTNULL"=FALSE, "MT_NULLLEFT"=FALSE, "MT_NULLCENTRE"=TRUE, "MT_STOPNULL"=FALSE, "MT_FILTERSWITCH"=TRUE}) -> ()  [unwired: 2 in, 2 out]
                    n167 = property on="AnalogInput" class="WFChart (strict)"("History Data"=dbl[] []) -> ()  [unwired: 2 in, 2 out]
                    n168 = property on="FStart" class="DigNum (strict)"("Value"=w294) -> ()  [unwired: 2 in, 2 out]
                    n169 = property on="MinLeft(0)" class="DigNum (strict)"("Value"=u16 0 ("MinLeft(0)")) -> ()  [unwired: 2 in, 2 out]
                    n170 = property on="MaxRight(1023)" class="DigNum (strict)"("Value"=u16 1023 ("MaxRight(1023)")) -> ()  [unwired: 2 in, 2 out]
                    n171 = call "CalculateMicrostepFrequency.vi"("div_i"=w276, "velocity"=w289, "clkdiv"=w269) -> ("f_microstep"=w293:dbl)
                    n172 = call "CalculateMicrostepFrequency.vi"("div_i"=w276, "velocity"=u16 100, "clkdiv"=w269) -> ("f_microstep"=w277:dbl)
                    n173 = property on="CurrentPosition" class="DigNum (strict)"("Value"=w301) -> ()  [unwired: 2 in, 2 out]
                    n174 = property on="CurrentActivity" class="Enum (strict)"("Value"=w301) -> ()  [unwired: 2 in, 2 out]
                    n175 = property on="FMin" class="DigNum (strict)"("Value"=w293) -> ()  [unwired: 2 in, 2 out]
                    n176 = call "GetUnitInformation.vi"("handle in"=w284, "UnitAddress(0)"=w285, "error in"=w283) -> ("handle out"=w287:i32, "FirmwareRevision"=w281:u8, "ResetFlag"=w280:u8, "Temperature"=w278:i16, "SerialNumber"=w282:u16, "error out"=w286:errorcluster)  [unwired: 11 in]
                    n177 = property on="Temperature" class="DigNum (strict)"("Value"=w278) -> ()  [unwired: 2 in, 2 out]
                    n178 = property on="SerialNumber" class="DigNum (strict)"("Value"=w282) -> ()  [unwired: 2 in, 2 out]
                    n179 = property on="FirmwareRevision" class="DigNum (strict)"("Value"=w281) -> ()  [unwired: 2 in, 2 out]
                    n180 = property on="StopFlag" class="Bool (strict)"("Value"=FALSE ("StopFlag")) -> ()  [unwired: 2 in, 2 out]
                    n181 = call "CalculateMicrostepFrequency.vi"("div_i"=w276, "velocity"=w288, "clkdiv"=w269) -> ("f_microstep"=w292:dbl)
                    n182 = Not Equal To 0?(x=w280) -> (x != 0?=w279:bool)
                    n183 = property on="ResetFlag" class="Bool (strict)"("Value"=w279) -> ()  [unwired: 2 in, 2 out]
                    n184 = property on="Fmax" class="DigNum (strict)"("Value"=w292) -> ()  [unwired: 2 in, 2 out]
                    n185 = property on="FRefMax" class="DigNum (strict)"("Value"=w277) -> ()  [unwired: 2 in, 2 out]
                  }
                  frame Error {
                  }
                }
              }
              event "Tab Control": Value Change {
                n186 = event-data() -> ("NewVal"=w313:T2)  [unwired: 1 in]
                n187 = case shown="\"Unit Info\"" w313 {
                  tunnel: w316 -> [_ _ _ _ _ w326 _ _ _ _]
                  tunnel: [_ _ _ _ _ w325 _ _ _ _] -> w318
                  tunnel: w315 -> [_ _ _ _ _ w319 _ _ _ _]
                  tunnel: w314 -> [_ _ _ _ _ _ _ _ _ _]
                  frame Default {
                  }
                  frame "Ramp" {
                  }
                  frame "MotorParameters" {
                  }
                  frame "Reference Search" {
                  }
                  frame "Current" {
                  }
                  frame "Unit Info" {
                    n188 = call "GetUnitInformation.vi"("handle in"=w326, "UnitAddress(0)"=w319) -> ("FirmwareRevision"=w324:u8, "ResetFlag"=w320:u8, "Temperature"=w323:i16, "SerialNumber"=w322:u16, "error out"=w325:errorcluster)  [unwired: 12 in, 1 out]
                    n189 = property on="FirmwareRevision" class="DigNum (strict)"("Value"=w324) -> ()  [unwired: 2 in, 2 out]
                    n190 = Not Equal To 0?(x=w320) -> (x != 0?=w321:bool)
                    n191 = property on="ResetFlag" class="Bool (strict)"("Value"=w321) -> ()  [unwired: 2 in, 2 out]
                    n192 = property on="Temperature" class="DigNum (strict)"("Value"=w323) -> ()  [unwired: 2 in, 2 out]
                    n193 = property on="SerialNumber" class="DigNum (strict)"("Value"=w322) -> ()  [unwired: 2 in, 2 out]
                  }
                  frame "Velocity" {
                  }
                  frame "Input" {
                  }
                  frame "LimitSwitch" {
                  }
                  frame "Interface" {
                  }
                }
                n194 = Equal?(x=w313, y=T2."Input") -> (x = y?=w317:bool)
              }
              event "PdcInt": Value Change {
                n195 = event-data() -> ("NewVal"=w330:i32)  [unwired: 1 in]
                n196 = property on="PdcInt" class="DigNum (strict)"("Value"=w330) -> ()  [unwired: 2 in, 2 out]
              }
              event "Stop": Value Change {
                n197 = event-data() -> ("NewVal"=w334:bool)  [unwired: 1 in]
              }
            }
            "error out" <- w69
            n198 = Select(t=i8 1, s=w69, f=i8 0) -> (s? t:f=→"error chart":i8)
          }
          n199 = call "ClosePort.vi"("handle"=w64) -> ()  [unwired: 19 in]
        }
        frame Error {
          n200 = case shown="False" w335 {
            tunnel: w336 -> [w337 _]
            frame False {
              n201 = call <vilib>:"Simple Error Handler.vi"("error in (no error)"=w337) -> ()  [unwired: 4 in, 5 out]
            }
            frame True {
            }
          }
        }
      }
    }
  }
